vi "Pie Page.vi"() -> ()   [LabVIEW 2017, in "3D Pie.lvclass"]
uses:
  <vilib>/Math Plots/3D Math Plots/3D Pie/3D Pie/3D Pie.lvclass
  <vilib>/Math Plots/3D Math Plots/3D Pie/3D Pie/Typedef/3D Pie Property Array.ctl
  <vilib>/Math Plots/3D Math Plots/3D Pie/3D Pie/Typedef/3D Pie Property.ctl
  <vilib>/Math Plots/3D Math Plots/3D Plot/3D Plot/Typedef/Line Type.ctl
  <vilib>/Math Plots/3D Math Plots/3D Plot/3D Plot/Typedef/Dialog State.ctl
  <vilib>/Math Plots/3D Math Plots/3D Plot/3D Plot/Typedef/Temp Scene State.ctl
  <vilib>/Math Plots/3D Math Plots/3D Plot/3D Plot/Typedef/Temp Scene Property Action.ctl
  <vilib>/Math Plots/3D Math Plots/3D Plot/3D Plot/3D Plot.lvclass
panel:
  in  "Label Color":u32(colorbox) caption="Label color"
  in  "Label Size":u16=1 caption="Label size" min=1 step=1
  in  "Color and Name":cluster{"Label Color":u32, "String":string}[](array[cluster]) caption="Color and name"
  in  "Label Mode":u16(ring) caption="Label mode" items=["None ", "Show Percentage", "Show String"]
  in  "Height":sgl=0.001 min=0.001 step=1
  in  "Show Offset":bool caption="Show offset"
  in  "Center X":sgl
  in  "Center Z":sgl
  in  "Center Y":sgl
  in  "Line Style":u16(ring) caption="Line style"
  in  "Antialiasing":bool
  in  "Line Width":sgl caption="Line width" min=0.001 step=1
  in  "Line Color":u32(colorbox) caption="Line color"
  out "Pie Property Out":T1
  in  "Pie Property In":T1
  in  "YZ Plane Projection":bool caption="YZ plane projection"
  in  "XZ Plane Projection":bool caption="XZ  plane projection"
  in  "XY Plane Projection":bool caption="XY  plane projection"
  in  "Coordinate System":u16(ring) caption="Coordinate system" items=["Cartesian", "Cylindrical", "Spherical"]
  in  "Plot Opacity":sgl(slide) caption="Plot opacity(%)" min=0 max=100 scale=0.0..100.0
  in  "Plot List":i32(listbox)
  in  "Move Down":bool
  in  "Move Up":bool
  in  "Delete":bool
  in  "New":bool
  in  "Event Registration":refnum<event-registration>
  # "Pie"
  # "General"
  # "Projection"
  # "Pie"
  # "Outline"
  # "Pie Cylinder"
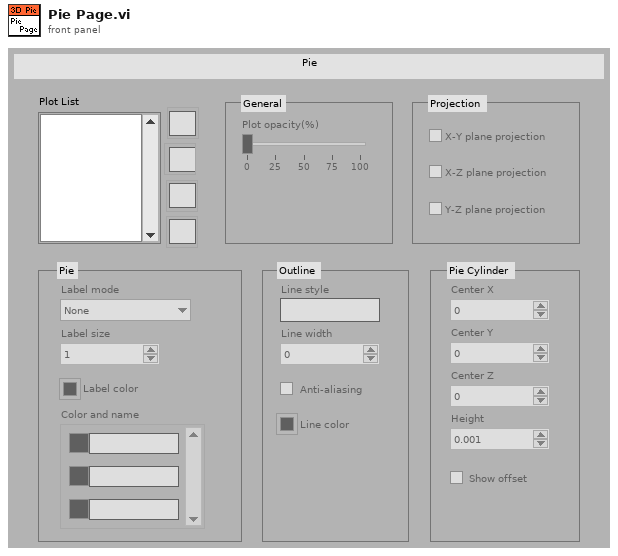
[diagram p1: front panel]
types:
  T1 = typedef "3D Pie.lvclass/3D Pie Property Array.ctl" = T2[]
  T2 = typedef "3D Pie.lvclass/3D Pie Property.ctl" = cluster{"General Property":cluster{"Plot Name":string, "Coordinate System":enum16{"Cartesian", "Cylindrical", "Spherical"}, "Opacity":sgl}, "Projection Property":cluster{"Draw XY":bool, "Draw YZ":bool, "Draw XZ":bool}, "Plot Property":cluster{"Line Style":T3, "Line Width":sgl, "Line Color":u32, "Antialiasing":bool}, "Pie Property":cluster{"Pie Height":sgl, "Pie Center":cluster{"X":sgl, "Y":sgl, "Z":sgl}, "Label Mode":enum16{"None", "Show Percentage", "Show String"}, "Label Size":u16, "Label Color":u32, "Color Pair Array":cluster{"Color":u32, "String":string}[], "Slice Offset?":bool}}
  T3 = typedef "3D Plot.lvclass/Line Type.ctl" = enum16{"None", "Solid", "Dash", "Dot", "Dash Dot"}
  T4 = typedef "3D Plot.lvclass/Dialog State.ctl" = enum16{"Initialize", "Read Porperty", "Write Property", "Idle", "Exit"}
  T5 = typedef "3D Plot.lvclass/Temp Scene State.ctl" = enum16{"Create", "Update Scene", "Get Plot Representation", "Destory"}
  T6 = typedef "3D Plot.lvclass/Temp Scene Property Action.ctl" = enum16{"Graph Property", "Light Property", "Axis Property", "Value Pair Property", "Format Property", "Cursor Property", "Plot Specific Property"}
  T7 = typedef "3D Plot.lvclass/Multiplot Representation.ctl" = cluster{"Plot Represention Array":T8[], "Max Range":T9}
  T8 = typedef "3D Plot.lvclass/Plot Representation.ctl" = cluster{"Plot ID":i32, "Plot Range":T9, "Mesh Data":T10, "Dimension":cluster{"X Dimension":i32, "Y Dimension":i32}, "Ramp Range":T9}
  T9 = typedef "3D Plot.lvclass/Range Clusters.ctl" = cluster{"X Range":cluster{"Max X":sgl, "Min X":sgl}, "Y Range":cluster{"Max Y":sgl, "Min Y":sgl}, "Z Range":cluster{"Max Z":sgl, "Min Z":sgl}}
  T10 = typedef "3D Plot.lvclass/Mesh Data.ctl" = cluster{"Index Array":u32[], "Vertex Array":cluster{"X":sgl, "Y":sgl, "Z":sgl}[], "Normal Array":cluster{"X":sgl, "Y":sgl, "Z":sgl}[], "Color Index Array":i32[]}
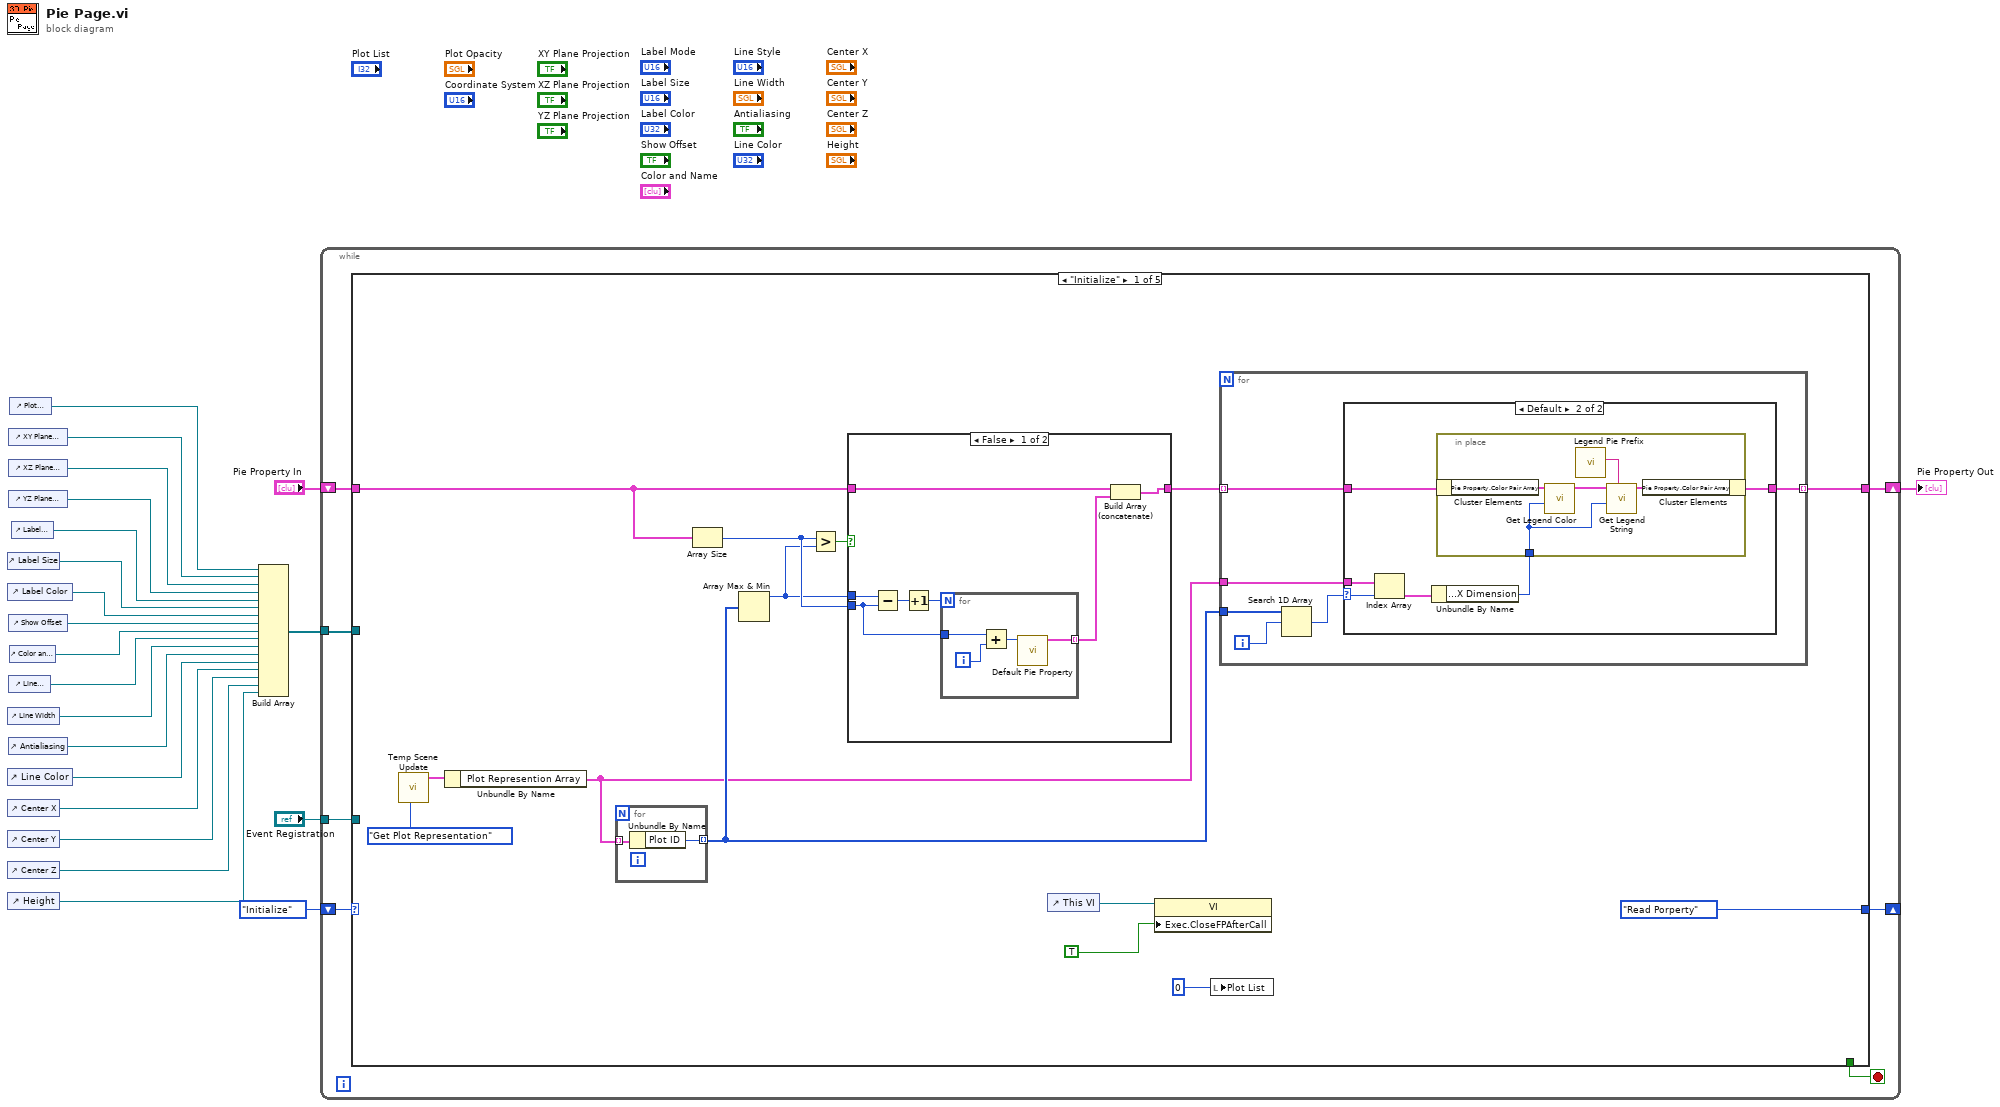
[diagram p0: block diagram]
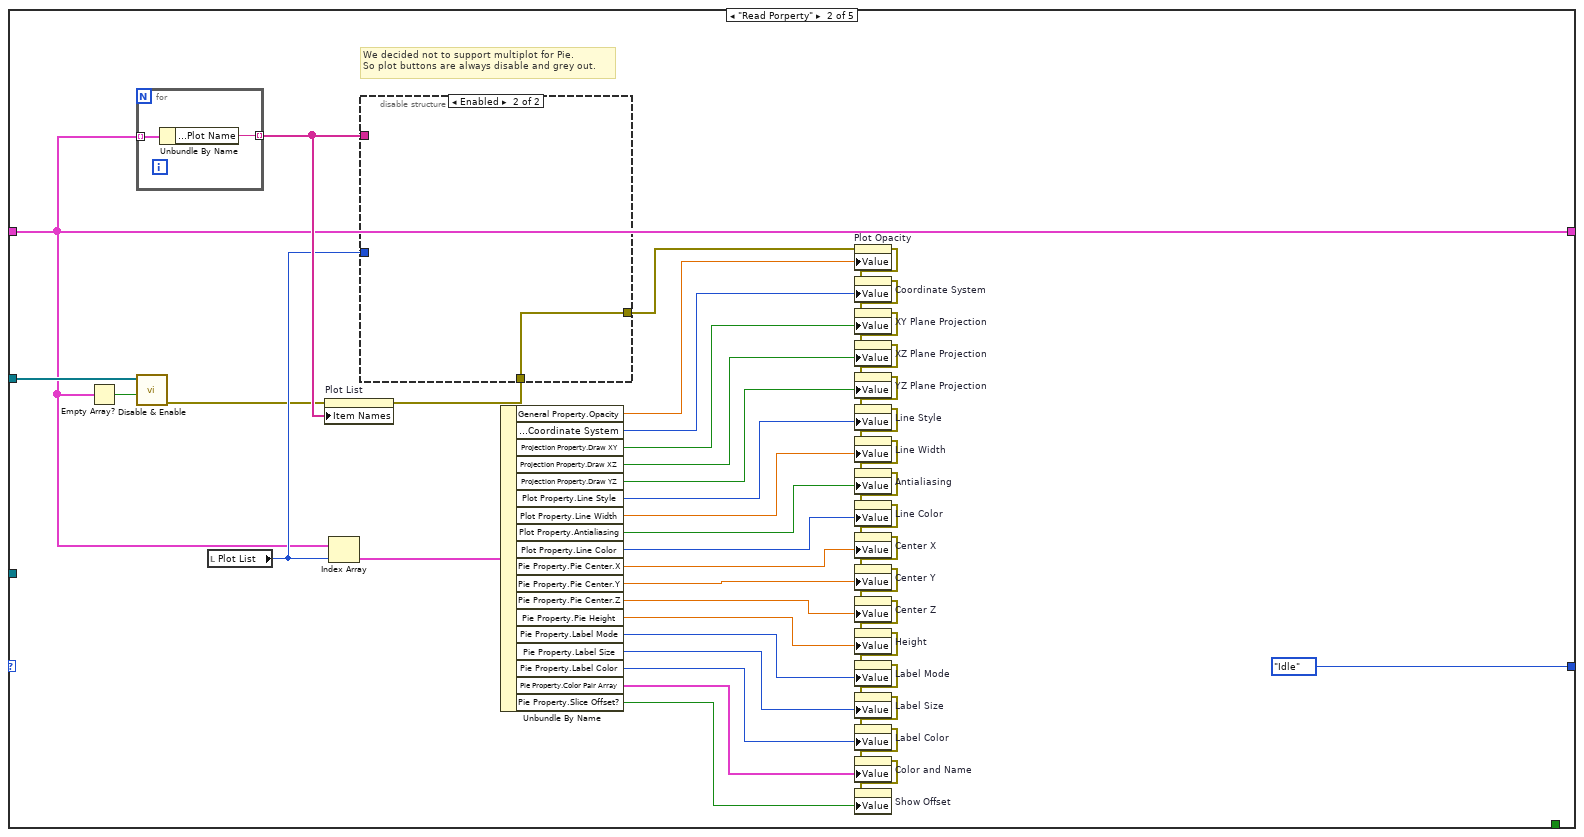
[diagram p4: hidden frame]
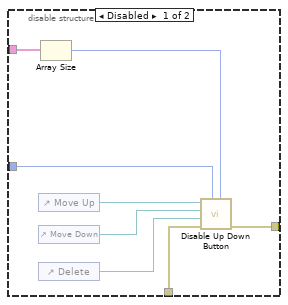
[diagram p5: hidden frame]
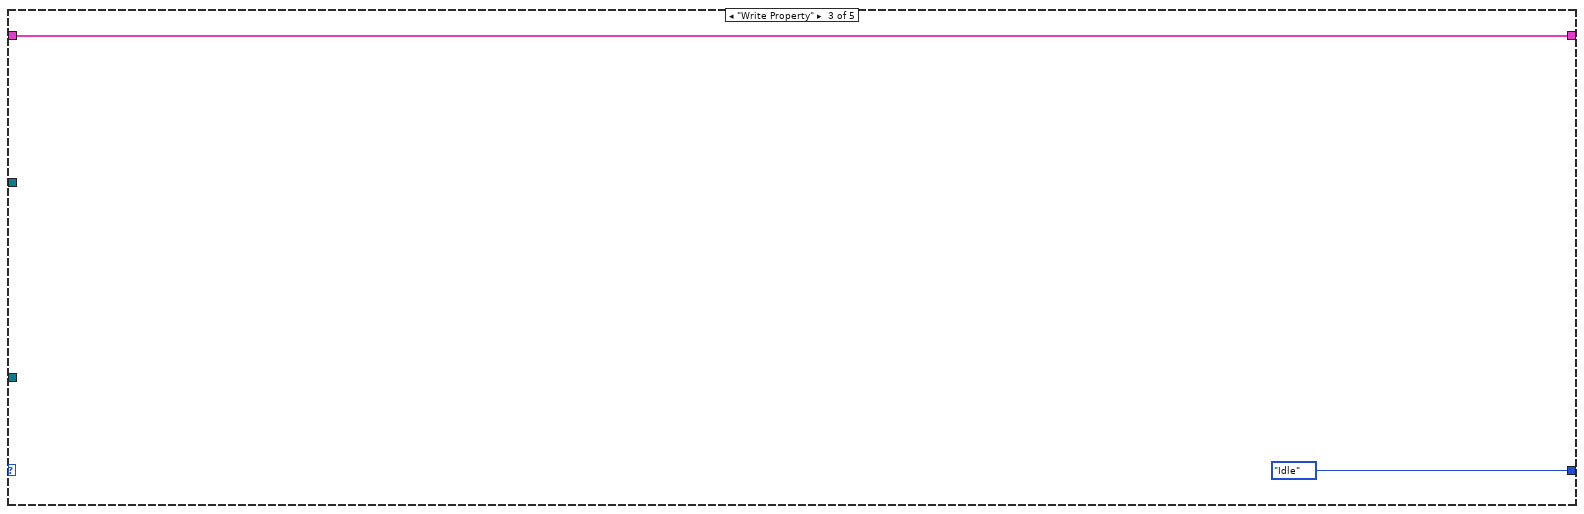
[diagram p6: hidden frame]
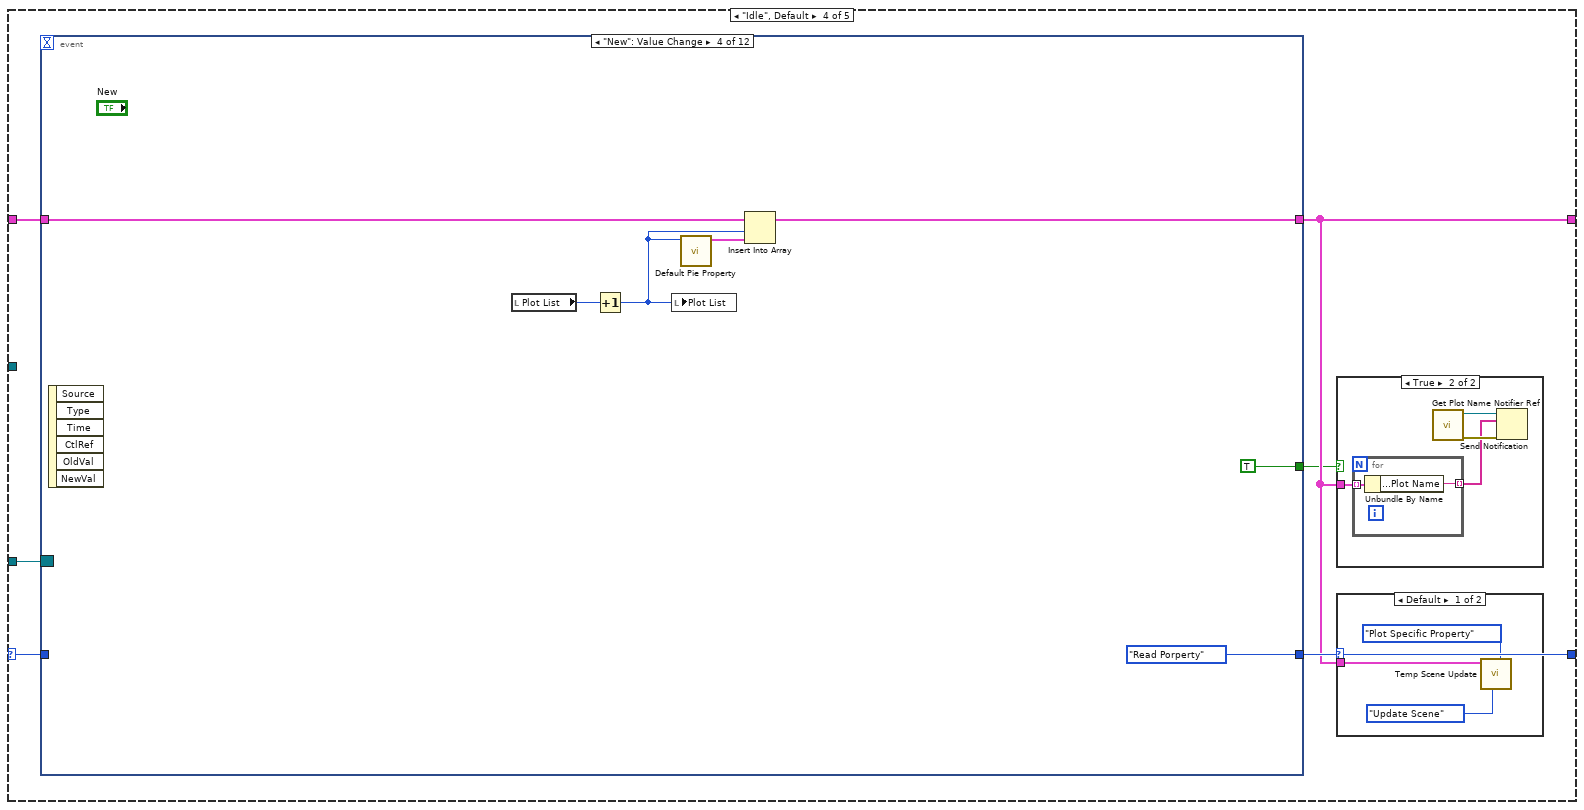
[diagram p7: hidden frame]
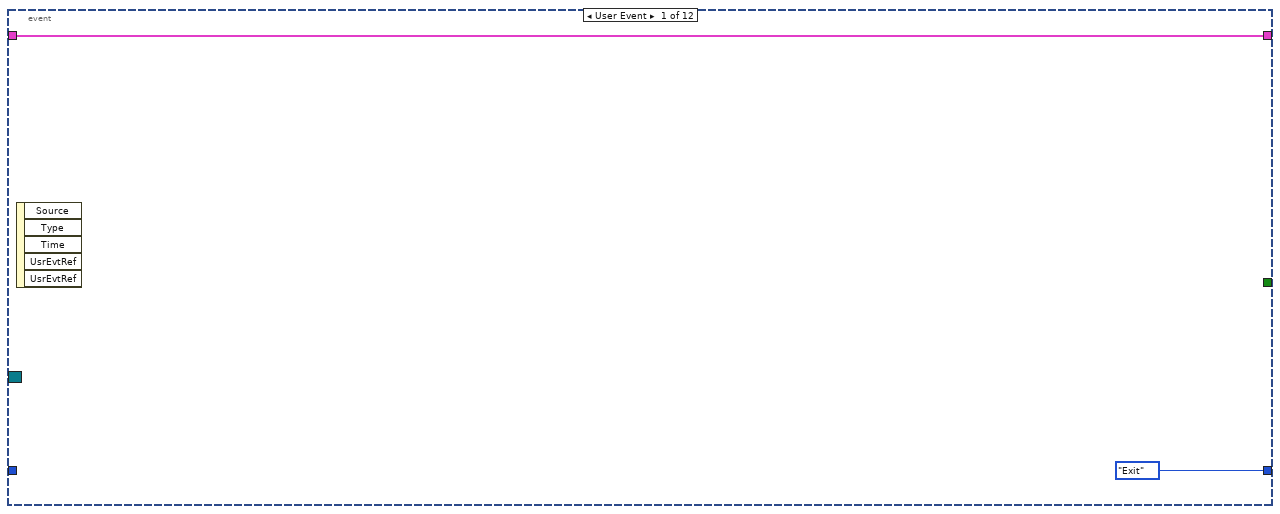
[diagram p10: hidden frame]
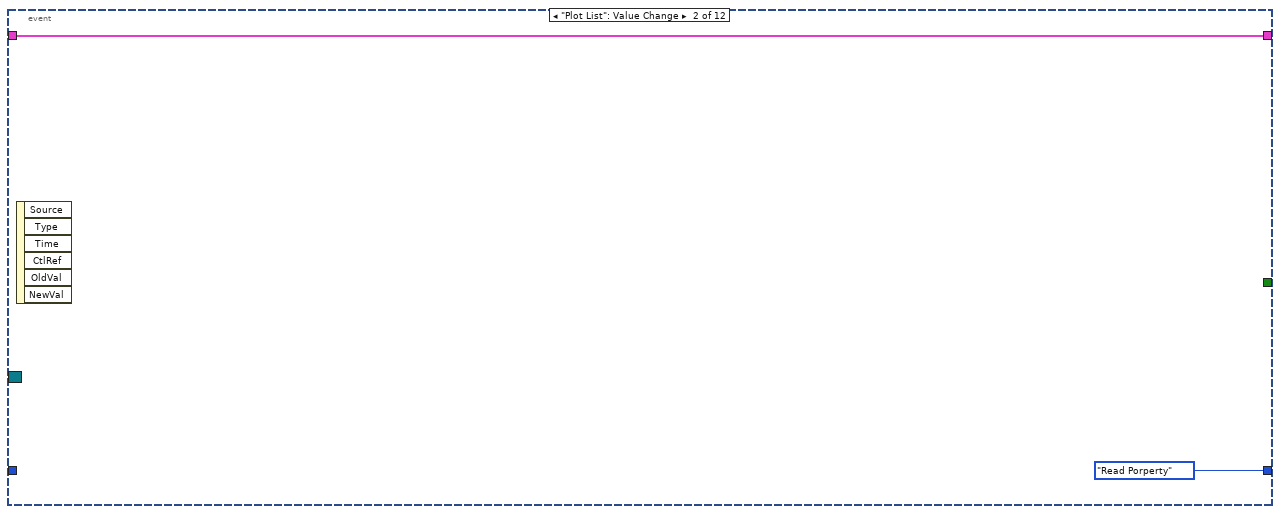
[diagram p11: hidden frame]
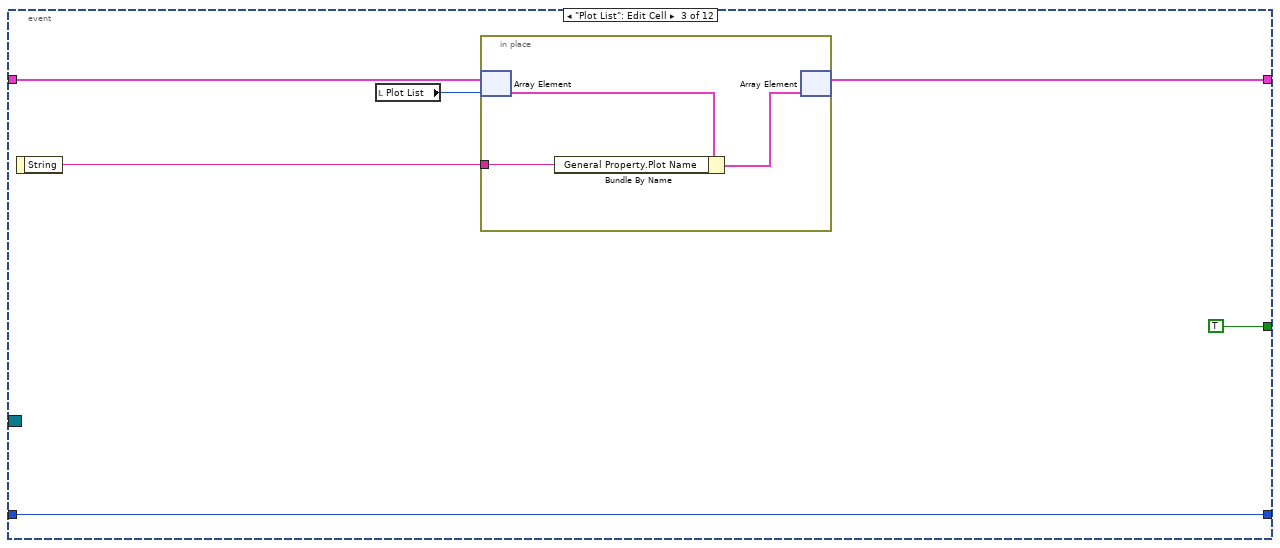
[diagram p12: hidden frame]
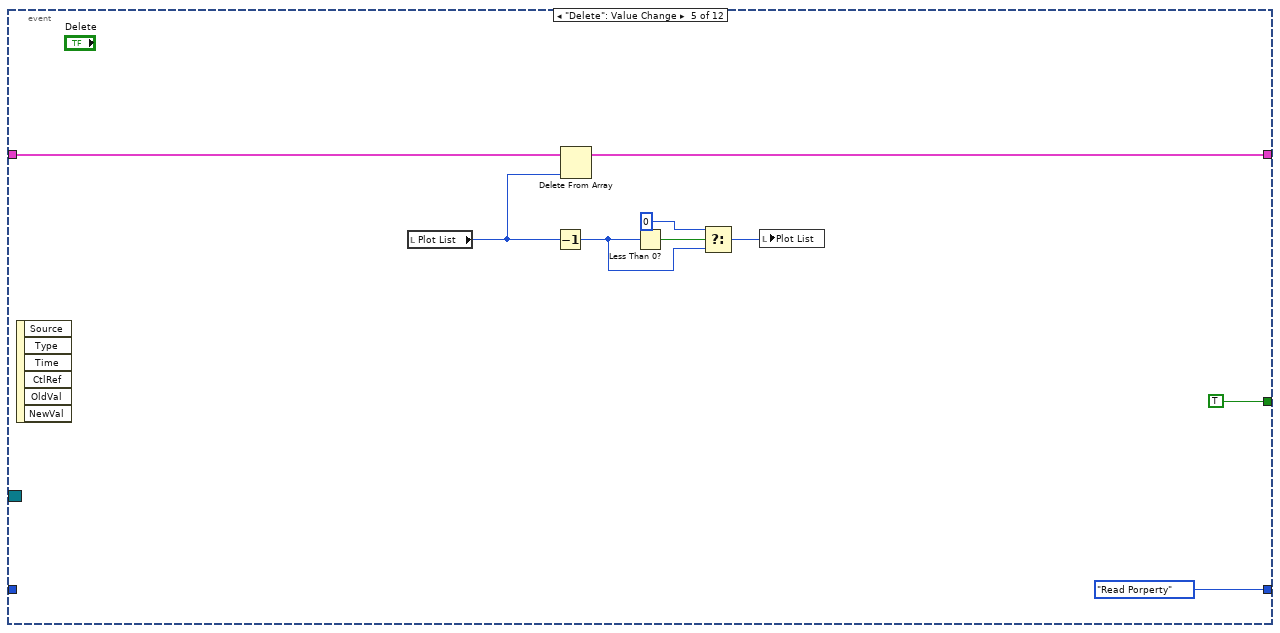
[diagram p13: hidden frame]
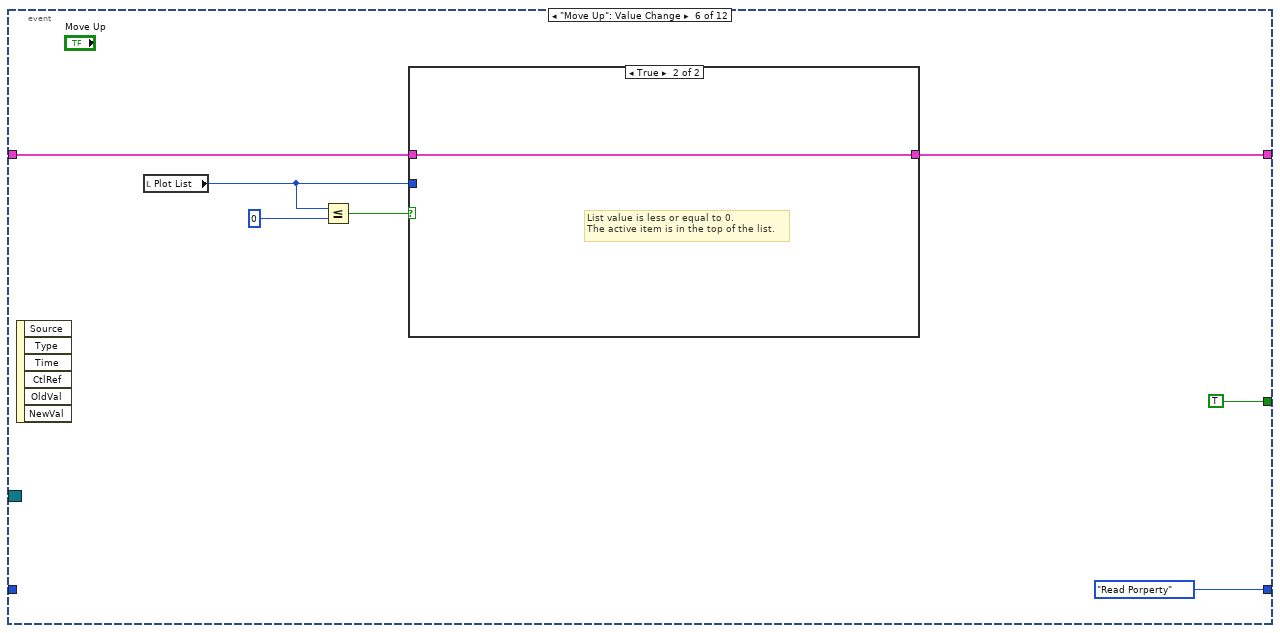
[diagram p14: hidden frame]
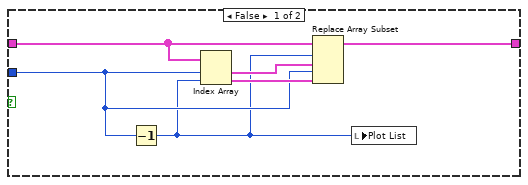
[diagram p15: hidden frame]
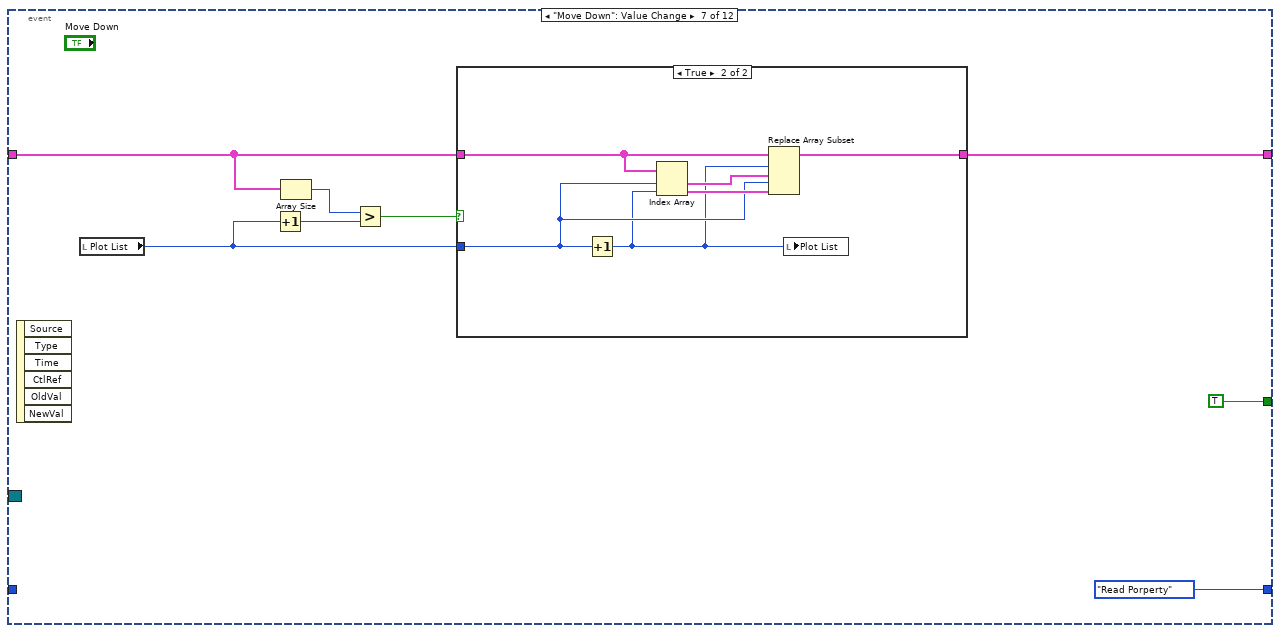
[diagram p16: hidden frame]
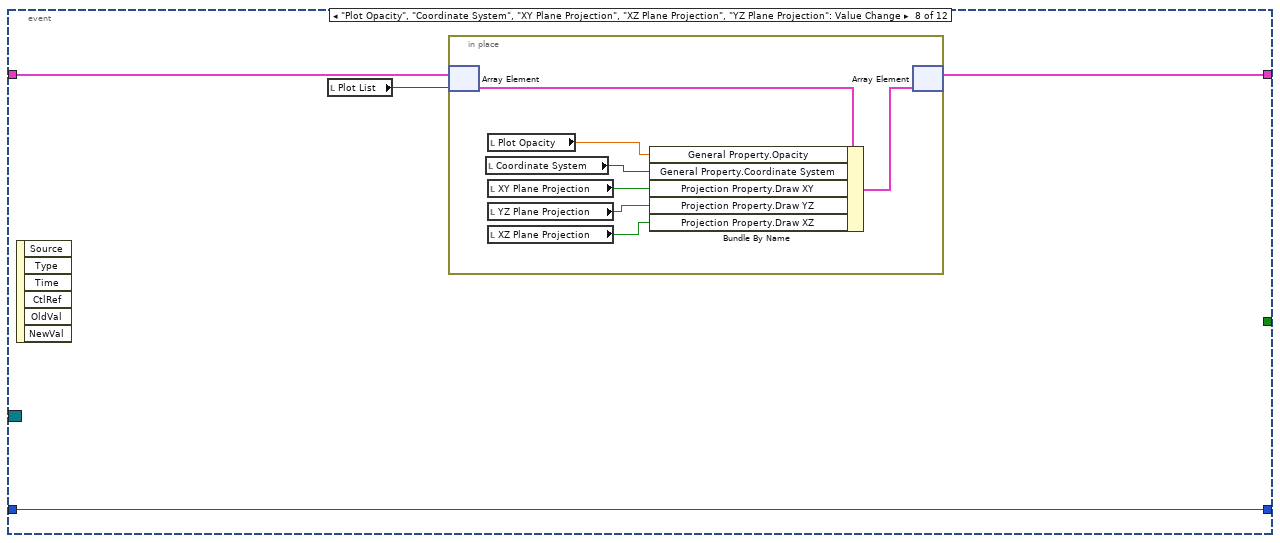
[diagram p18: hidden frame]
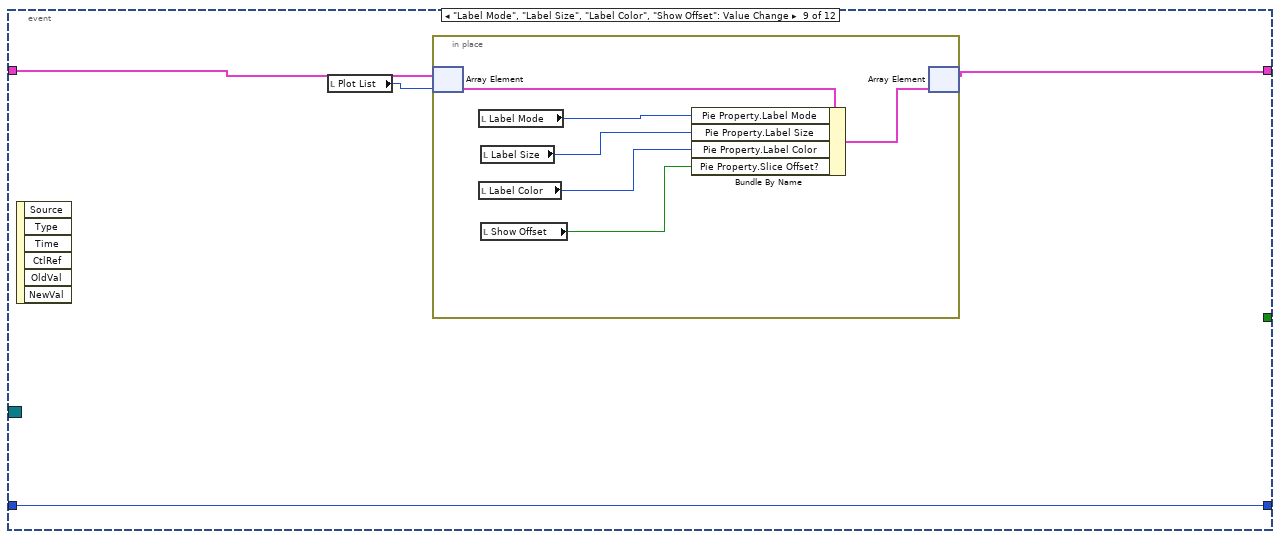
[diagram p19: hidden frame]
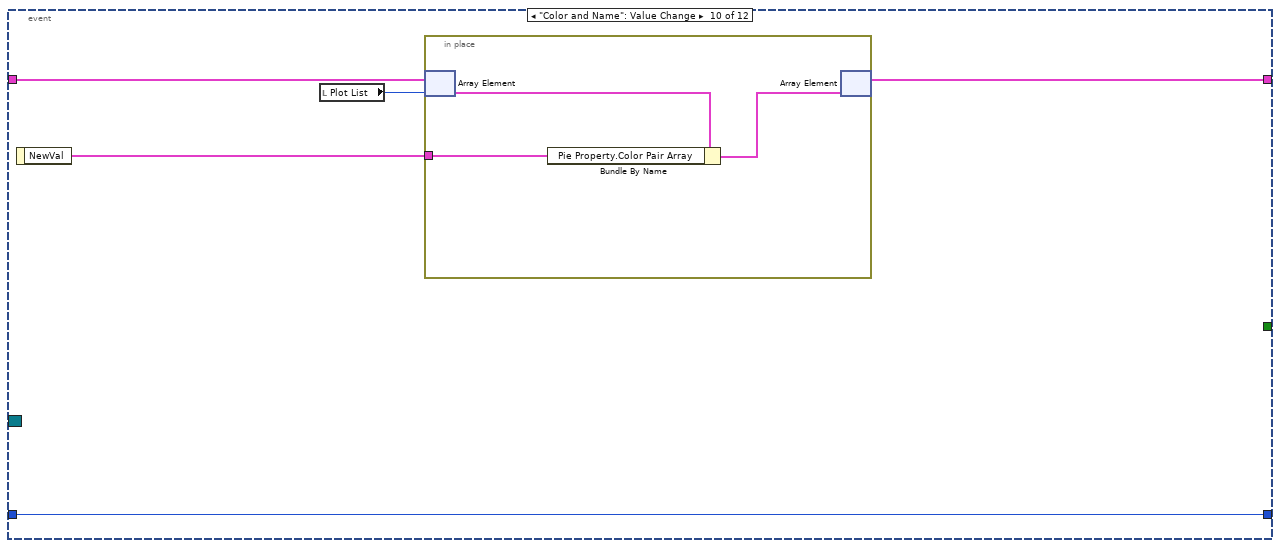
[diagram p20: hidden frame]
diagram:
  n1 = control-ref of="Label Size"() -> (w13:refnum<vi>)
  n2 = control-ref of="Label Color"() -> (w12:refnum<vi>)
  n3 = control-ref of="Line Width"() -> (w8:refnum<vi>)
  n4 = control-ref of="Line Color"() -> (w6:refnum<vi>)
  n5 = control-ref of="Center X"() -> (w5:refnum<vi>)
  n6 = control-ref of="Center Y"() -> (w4:refnum<vi>)
  n7 = control-ref of="Center Z"() -> (w3:refnum<vi>)
  n8 = control-ref of="Height"() -> (w2:refnum<vi>)
  n9 = control-ref of="XY Plane Projection"() -> (w17:refnum<vi>)
  n10 = control-ref of="XZ Plane Projection"() -> (w16:refnum<vi>)
  n11 = control-ref of="YZ Plane Projection"() -> (w15:refnum<vi>)
  n12 = control-ref of="Show Offset"() -> (w11:refnum<vi>)
  n13 = control-ref of="Line Style"() -> (w9:refnum<vi>)
  n14 = control-ref of="Antialiasing"() -> (w7:refnum<vi>)
  n15 = control-ref of="Plot Opacity"() -> (w18:refnum<vi>)
  n16 = control-ref of="Color and Name"() -> (w10:refnum<vi>)
  n17 = control-ref of="Label Mode"() -> (w14:refnum<vi>)
  n18 = Build Array(w18, w17, w16, w15, w14, w13, w12, w11, w10, w9, w8, w7, w6, w5, w4, w3, w2) -> (w1:refnum<vi>[])
  n19 = while {
    shift-right: [w28] -> w19
    shift-left: "Pie Property In" -> [w29]
    shift-right: [w24] -> _
    shift-left: Dialog_State."Initialize" -> [w27]
    tunnel: "Event Registration" -> [w25]
    tunnel: w1 -> [w23]
    stop <- w26 stop-if-true
    n20 = case shown="\"Initialize\"" w27 {
      selector: w27 -> [_ _ _ w137 _]
      tunnel: w29 -> [w34 w113 w132 w139 w256]
      tunnel: [w39 w113 w132 w135 w256] -> w28
      tunnel: [Dialog_State."Read Porperty" Dialog_State."Idle" Dialog_State."Idle" w136 Dialog_State."Exit"] -> w24
      tunnel: [_ _ _ _ TRUE] -> w26
      tunnel: w25 -> [_ _ _ w138 _]
      tunnel: w23 -> [_ w114 _ _ _]
      frame "Initialize" {
        n21 = call <vilib>:"Temp Scene Update.vi"("State"=Temp_Scene_State."Get Plot Representation") -> ("Multiplot Representation"=w31:T7)  [unwired: 5 in, 5 out]
        n22 = Unbundle By Name(w31) -> ("Plot Represention Array"=w30:T8[])
        n23 = for {
          tunnel: w30 -> [w57] mode=indexing
          tunnel: [w56] -> w32 mode=indexing
          n24 = Unbundle By Name(w57) -> ("Plot ID"=w56:i32)
        }
        n25 = Array Size(array=w34) -> (size(s)=w36:i32)
        n26 = Array Max & Min(array=w32) -> (max value=w35:i32)  [unwired: 3 out]
        n27 = Greater?(x=w36, y=w35) -> (0:w37:bool)
        n28 = case shown="False" w37 {
          tunnel: [w48 w55] -> w33
          tunnel: w34 -> [w50 w55]
          tunnel: w36 -> [w44 _]
          tunnel: w35 -> [w45 _]
          frame False {
            n29 = Subtract(x=w45, y=w44) -> (x-y=w47:i32)
            n30 = Increment(x=w47) -> (x+1=w46:i32)
            n31 = for {
              N: w46 -> [_]
              tunnel: w44 -> [w53]
              tunnel: [w51] -> w49 mode=indexing
              i -> [w54]
              n32 = Add(x=w53, y=w54) -> (x+y=w52:i32)
              n33 = call <vilib>:"Default Pie Property.vi"("Plot ID"=w52) -> ("Default Property"=w51:T2)  [unwired: 10 out]
            }
            n34 = Build Array (concatenate)(w50, w49) -> (w48:T1)
          }
          frame True {
          }
        }
        n35 = control-ref of="This VI"() -> (w42:refnum<vi>)
        n36 = property class="VI"(reference=w42, "Exec.CloseFPAfterCall"=TRUE ("Execution:Close After Call")) -> ()  [unwired: 1 in, 2 out]
        n37 = local write "Plot List"(0 ("Plot List")) -> ()
        n38 = for {
          tunnel: w33 -> [w63] mode=indexing
          tunnel: w30 -> [w61]
          tunnel: [w62] -> w39 mode=indexing
          tunnel: w32 -> [w60]
          i -> [w59]
          n39 = Search 1D Array(1D array=w60, element=w59) -> (index of element=w58:i32)  [unwired: 1 out]
          n40 = case shown="Default" w58 {
            selector: w58 -> [_ w65]
            tunnel: w63 -> [w64 w69]
            tunnel: [w64 w68] -> w62
            tunnel: w61 -> [_ w67]
            frame -1 {
            }
            frame Default {
              n41 = Index Array(array=w67, index=w65) -> (element=w66:T8)
              n42 = Unbundle By Name(w66) -> ("Dimension.X Dimension"=w70:i32)
              n43 = in-place {
                in-place-border: w70 -> [w71]
                n44 = in-place-cluster #1(w69) -> ("Pie Property.Color Pair Array"=w73:cluster{"Color":u32, "String":string}[])
                n45 = call <vilib>:"Get Legend Color.vi"("Pair Array Length"=w71, "Color Pair Array In"=w73) -> ("Color Pair Array Out"=w75:cluster{"Color":u32, "String":string}[])  [unwired: 9 out]
                n46 = call <vilib>:"Legend Pie Prefix.vi"() -> ("Prefix Out"=w74:string)  [unwired: 11 out]
                n47 = call <vilib>:"Get Legend String.vi"("Initial String"=w74, "Pair Array Length"=w71, "Color Pair Array In"=w75) -> ("Color Pair Array Out"=w72:cluster{"Color":u32, "String":string}[])  [unwired: 8 out]
                n48 = in-place-cluster #1("Pie Property.Color Pair Array"=w72) -> (w68:T2)
              }
            }
          }
        }
      }
      frame "Read Porperty" {
        # "We decided not to support multiplot for Pie.\nSo plot buttons are always disable and grey out."
        n49 = Empty Array?(array=w113) -> (empty?=w115:bool)
        n50 = for {
          tunnel: w113 -> [w131] mode=indexing
          tunnel: [w130] -> w118 mode=indexing
          n51 = Unbundle By Name(w131) -> ("General Property.Plot Name"=w130:string)
        }
        n52 = call <vilib>:"Disable & Enable.vi"("Disabled?"=w115, "Control Ref Array"=w114) -> ("error out"=w112:errorcluster)  [unwired: 1 in, 8 out]
        n53 = local read "Plot List"() -> (w116:i32)
        n54 = property on="Plot List" class="LstBox (strict)"(error in=w112, "Item Names"=w118) -> (error out=w117:errorcluster)  [unwired: 1 in, 1 out]
        n55 = Index Array(array=w113, index=w116) -> (element=w119:T2)
        n56 = disable-structure shown="Enabled" {
          disable-tunnel: w118 -> [w124 _]
          disable-tunnel: w117 -> [w123 w129]
          disable-tunnel: w116 -> [w122 _]
          disable-tunnel: [w121 w129] -> w76
          frame Disabled {
            n57 = control-ref of="Move Up"() -> (w126:refnum<vi>)
            n58 = control-ref of="Move Down"() -> (w127:refnum<vi>)
            n59 = control-ref of="Delete"() -> (w128:refnum<vi>)
            n60 = Array Size(array=w124) -> (size(s)=w125:i32)
            n61 = call <vilib>:"Disable Up Down Button.vi"("Length"=w125, "Index"=w122, "error in (no error)"=w123, "Delete Ref"=w128, "Move Down Ref"=w127, "Move Up Ref"=w126) -> ("error out"=w121:errorcluster)  [unwired: 5 out]
          }
          frame Enabled {
          }
        }
        n62 = Unbundle By Name(w119) -> ("General Property.Opacity"=w96:sgl, "General Property.Coordinate System"=w95:enum16{"Cartesian", "Cylindrical", "Spherical"}, "Projection Property.Draw XY"=w94:bool, "Projection Property.Draw XZ"=w93:bool, "Projection Property.Draw YZ"=w92:bool, "Plot Property.Line Style"=w91:T3, "Plot Property.Line Width"=w90:sgl, "Plot Property.Antialiasing"=w89:bool, "Plot Property.Line Color"=w88:u32, "Pie Property.Pie Center.X"=w87:sgl, "Pie Property.Pie Center.Y"=w86:sgl, "Pie Property.Pie Center.Z"=w85:sgl, "Pie Property.Pie Height"=w79:sgl, "Pie Property.Label Mode"=w84:enum16{"None", "Show Percentage", "Show String"}, "Pie Property.Label Size"=w83:u16, "Pie Property.Label Color"=w82:u32, "Pie Property.Color Pair Array"=w81:cluster{"Color":u32, "String":string}[], "Pie Property.Slice Offset?"=w80:bool)
        n63 = property on="Plot Opacity" class="Slide (strict)"(error in=w76, "Value"=w96) -> (error out=w111:errorcluster)  [unwired: 1 in, 1 out]
        n64 = property on="Coordinate System" class="Ring (strict)"(error in=w111, "Value"=w95) -> (error out=w110:errorcluster)  [unwired: 1 in, 1 out]
        n65 = property on="XY Plane Projection" class="Bool (strict)"(error in=w110, "Value"=w94) -> (error out=w109:errorcluster)  [unwired: 1 in, 1 out]
        n66 = property on="XZ Plane Projection" class="Bool (strict)"(error in=w109, "Value"=w93) -> (error out=w108:errorcluster)  [unwired: 1 in, 1 out]
        n67 = property on="YZ Plane Projection" class="Bool (strict)"(error in=w108, "Value"=w92) -> (error out=w107:errorcluster)  [unwired: 1 in, 1 out]
        n68 = property on="Line Style" class="Ring (strict)"(error in=w107, "Value"=w91) -> (error out=w106:errorcluster)  [unwired: 1 in, 1 out]
        n69 = property on="Line Width" class="DigNum (strict)"(error in=w106, "Value"=w90) -> (error out=w105:errorcluster)  [unwired: 1 in, 1 out]
        n70 = property on="Antialiasing" class="Bool (strict)"(error in=w105, "Value"=w89) -> (error out=w104:errorcluster)  [unwired: 1 in, 1 out]
        n71 = property on="Line Color" class="ColBox"(error in=w104, "Value"=w88) -> (error out=w103:errorcluster)  [unwired: 1 in, 1 out]
        n72 = property on="Center X" class="DigNum (strict)"(error in=w103, "Value"=w87) -> (error out=w102:errorcluster)  [unwired: 1 in, 1 out]
        n73 = property on="Center Y" class="DigNum (strict)"(error in=w102, "Value"=w86) -> (error out=w101:errorcluster)  [unwired: 1 in, 1 out]
        n74 = property on="Center Z" class="DigNum (strict)"(error in=w101, "Value"=w85) -> (error out=w78:errorcluster)  [unwired: 1 in, 1 out]
        n75 = property on="Height" class="DigNum (strict)"(error in=w78, "Value"=w79) -> (error out=w77:errorcluster)  [unwired: 1 in, 1 out]
        n76 = property on="Label Mode" class="Ring (strict)"(error in=w77, "Value"=w84) -> (error out=w100:errorcluster)  [unwired: 1 in, 1 out]
        n77 = property on="Label Size" class="DigNum (strict)"(error in=w100, "Value"=w83) -> (error out=w97:errorcluster)  [unwired: 1 in, 1 out]
        n78 = property on="Label Color" class="ColBox"(error in=w97, "Value"=w82) -> (error out=w98:errorcluster)  [unwired: 1 in, 1 out]
        n79 = property on="Color and Name" class="Arr (strict)"(error in=w98, "Value"=w81) -> (error out=w99:errorcluster)  [unwired: 1 in, 1 out]
        n80 = property on="Show Offset" class="Bool (strict)"(error in=w99, "Value"=w80) -> ()  [unwired: 1 in, 2 out]
      }
      frame "Write Property" {
      }
      frame "Idle", Default {
        n81 = event shown="[3] \"New\": Value Change" {
          selector: w138 -> [_ _ _ _ _ _ _ _ _ _ _ _]
          dyn-events: _ -> [_ _ _ _ _ _ _ _ _ _ _ _]
          timeout: _ -> [_ _ _ _ _ _ _ _ _ _ _ _]
          tunnel: w139 -> [w150 w152 w156 w166 w175 w180 w194 w208 w219 w232 w237 w247]
          tunnel: [w150 w152 w155 w165 w176 w179 w193 w207 w218 w231 w236 w246] -> w135
          tunnel: [Dialog_State."Exit" Dialog_State."Read Porperty" w154 Dialog_State."Read Porperty" Dialog_State."Read Porperty" Dialog_State."Read Porperty" Dialog_State."Read Porperty" w210 w221 w228 w239 w248] -> w136
          tunnel: w137 -> [_ _ w154 _ _ _ _ w210 w221 w228 w239 w248]
          tunnel: [_ _ TRUE TRUE TRUE TRUE TRUE _ _ _ _ _] -> w134
          event User Event {
            n82 = event-data() -> ()  [unwired: 6 out]
          }
          event "Plot List": Value Change {
            n83 = event-data() -> ()  [unwired: 7 out]
          }
          event "Plot List": Edit Cell {
            n84 = event-data() -> ("String"=w157:string)  [unwired: 1 out]
            n85 = local read "Plot List"() -> (w158:i32)
            n86 = in-place {
              in-place-border: w157 -> [w159]
              n87 = in-place-array #2(w156, w158) -> (w161:T2)
              n88 = Bundle By Name(cluster=w161, "General Property.Plot Name"=w159) -> (w160:T2)
              n89 = in-place-array #2(w160) -> (w155:T1)  [unwired: 1 out]
            }
          }
          event "New": Value Change {
            n90 = event-data() -> ()  [unwired: 7 out]
            n91 = local read "Plot List"() -> (w167:i32)
            n92 = Increment(x=w167) -> (x+1=w163:i32)
            n93 = local write "Plot List"(w163) -> ()
            n94 = call <vilib>:"Default Pie Property.vi"("Plot ID"=w163) -> ("Default Property"=w162:T2)  [unwired: 10 out]
            n95 = Insert Into Array(array=w166, index=w163, new element=w162) -> (w165:T1)
          }
          event "Delete": Value Change {
            n96 = event-data() -> ()  [unwired: 7 out]
            n97 = local read "Plot List"() -> (w171:i32)
            n98 = Decrement(x=w171) -> (x-1=w172:i32)
            n99 = Delete From Array(array=w175, index=w171) -> (array with subset deleted=w176:T1)  [unwired: 1 in, 1 out]
            n100 = Less Than 0?(x=w172) -> (x < 0?=w174:bool)
            n101 = Select(t=0, s=w174, f=w172) -> (s? t:f=w170:i32)
            n102 = local write "Plot List"(w170) -> ()
          }
          event "Move Up": Value Change {
            n103 = event-data() -> ()  [unwired: 7 out]
            n104 = local read "Plot List"() -> (w181:i32)
            n105 = Less Or Equal?(x=w181, y=0) -> (x <= y?=w182:bool)
            n106 = case shown="True" w182 {
              tunnel: w180 -> [w188 w191]
              tunnel: [w187 w191] -> w179
              tunnel: w181 -> [w186 _]
              frame False {
                n107 = Decrement(x=w186) -> (x-1=w185:i32)
                n108 = Index Array(array=w188, index #1=w186, index #2=w185) -> (element #1=w190:T2, element #2=w189:T2)
                n109 = Replace Array Subset(array=w188, new element #1=w190, index #1=w185, new element #2=w189, index #2=w186) -> (w187:T1)
                n110 = local write "Plot List"(w185) -> ()
              }
              frame True {
                # "List value is less or equal to 0.\nThe active item is in the top of the list."
              }
            }
          }
          event "Move Down": Value Change {
            n111 = event-data() -> ()  [unwired: 7 out]
            n112 = local read "Plot List"() -> (w195:i32)
            n113 = Increment(x=w195) -> (x+1=w197:i32)
            n114 = Array Size(array=w194) -> (size(s)=w196:i32)
            n115 = Greater?(x=w196, y=w197) -> (0:w198:bool)
            n116 = case shown="True" w198 {
              tunnel: w194 -> [w200 w204]
              tunnel: [w200 w203] -> w193
              tunnel: w195 -> [_ w202]
              frame False {
                # "List value +1 is not less array length.\nThe active item is in the buttom of the list."
              }
              frame True {
                n117 = Increment(x=w202) -> (x+1=w201:i32)
                n118 = Index Array(array=w204, index #1=w202, index #2=w201) -> (element #1=w206:T2, element #2=w205:T2)
                n119 = Replace Array Subset(array=w204, new element #1=w206, index #1=w201, new element #2=w205, index #2=w202) -> (w203:T1)
                n120 = local write "Plot List"(w201) -> ()
              }
            }
          }
          event "Plot Opacity", "Coordinate System", "XY Plane Projection", "XZ Plane Projection", "YZ Plane Projection": Value Change {
            n121 = event-data() -> ()  [unwired: 7 out]
            n122 = local read "Plot List"() -> (w209:i32)
            n123 = in-place {
              n124 = in-place-array #3(w208, w209) -> (w213:T2)
              n125 = local read "Coordinate System"() -> (w211:u16)
              n126 = local read "Plot Opacity"() -> (w217:sgl)
              n127 = local read "XY Plane Projection"() -> (w216:bool)
              n128 = local read "YZ Plane Projection"() -> (w214:bool)
              n129 = local read "XZ Plane Projection"() -> (w215:bool)
              n130 = Bundle By Name(cluster=w213, "General Property.Opacity"=w217, "General Property.Coordinate System"=w211, "Projection Property.Draw XY"=w216, "Projection Property.Draw YZ"=w214, "Projection Property.Draw XZ"=w215) -> (w212:T2)
              n131 = in-place-array #3(w212) -> (w207:T1)  [unwired: 1 out]
            }
          }
          event "Label Mode", "Label Size", "Label Color", "Show Offset": Value Change {
            n132 = event-data() -> ()  [unwired: 7 out]
            n133 = local read "Plot List"() -> (w220:i32)
            n134 = in-place {
              n135 = in-place-array #4(w219, w220) -> (w224:T2)
              n136 = local read "Label Mode"() -> (w227:u16)
              n137 = local read "Label Color"() -> (w225:u32)
              n138 = local read "Label Size"() -> (w226:u16)
              n139 = local read "Show Offset"() -> (w222:bool)
              n140 = Bundle By Name(cluster=w224, "Pie Property.Label Mode"=w227, "Pie Property.Label Size"=w226, "Pie Property.Label Color"=w225, "Pie Property.Slice Offset?"=w222) -> (w223:T2)
              n141 = in-place-array #4(w223) -> (w218:T1)  [unwired: 1 out]
            }
          }
          event "Color and Name": Value Change {
            n142 = event-data() -> ("NewVal"=w230:cluster{"Label Color":u32, "String":string}[])  [unwired: 1 out]
            n143 = local read "Plot List"() -> (w229:i32)
            n144 = in-place {
              in-place-border: w230 -> [w233]
              n145 = in-place-array #5(w232, w229) -> (w235:T2)
              n146 = Bundle By Name(cluster=w235, "Pie Property.Color Pair Array"=w233) -> (w234:T2)
              n147 = in-place-array #5(w234) -> (w231:T1)  [unwired: 1 out]
            }
          }
          event "Line Style", "Line Width", "Antialiasing", "Line Color": Value Change {
            n148 = event-data() -> ()  [unwired: 7 out]
            n149 = local read "Plot List"() -> (w238:i32)
            n150 = in-place {
              n151 = in-place-array #6(w237, w238) -> (w242:T2)
              n152 = local read "Line Style"() -> (w245:u16)
              n153 = local read "Antialiasing"() -> (w243:bool)
              n154 = local read "Line Color"() -> (w240:u32)
              n155 = local read "Line Width"() -> (w244:sgl)
              n156 = Bundle By Name(cluster=w242, "Plot Property.Line Style"=w245, "Plot Property.Line Width"=w244, "Plot Property.Antialiasing"=w243, "Plot Property.Line Color"=w240) -> (w241:T2)
              n157 = in-place-array #6(w241) -> (w236:T1)  [unwired: 1 out]
            }
          }
          event "Center X", "Center Y", "Center Z", "Height": Value Change {
            n158 = event-data() -> ()  [unwired: 7 out]
            n159 = local read "Plot List"() -> (w249:i32)
            n160 = in-place {
              n161 = in-place-array #7(w247, w249) -> (w255:T2)
              n162 = local read "Height"() -> (w250:sgl)
              n163 = local read "Center X"() -> (w251:sgl)
              n164 = local read "Center Y"() -> (w253:sgl)
              n165 = local read "Center Z"() -> (w252:sgl)
              n166 = Bundle By Name(cluster=w255, "Pie Property.Pie Center.X"=w251, "Pie Property.Pie Center.Y"=w253, "Pie Property.Pie Center.Z"=w252, "Pie Property.Pie Height"=w250) -> (w254:T2)
              n167 = in-place-array #7(w254) -> (w246:T1)  [unwired: 1 out]
            }
          }
        }
        n168 = case shown="True" w134 {
          tunnel: w135 -> [_ w140]
          frame False {
          }
          frame True {
            n169 = for {
              tunnel: w140 -> [w145] mode=indexing
              tunnel: [w144] -> w141 mode=indexing
              n170 = Unbundle By Name(w145) -> ("General Property.Plot Name"=w144:string)
            }
            n171 = call <vilib>:"Get Plot Name Notifier Ref.vi"() -> ("error out"=w143:errorcluster, "Plot Names Notifier Ref"=w142:refnum<notifier>)  [unwired: 1 in, 9 out]
            n172 = Send Notification(notification=w141, notifier=w142, error in (no error)=w143) -> ()  [unwired: 2 out]
          }
        }
        n173 = case shown="Default" w136 {
          tunnel: w135 -> [w148 _]
          frame Default {
            n174 = call <vilib>:"Temp Scene Update.vi"("Property Name"=Temp_Scene_Property_Action."Plot Specific Property", "State"=Temp_Scene_State."Update Scene", "Property In"=w148) -> ()  [unwired: 3 in, 6 out]
          }
          frame "Exit" {
          }
        }
      }
      frame "Exit" {
      }
    }
  }
  "Pie Property Out" <- w19
